vi "Calculate Average Center.vi"(11 "Gantry Fiducials":dbl[](array[numeric])) -> (3 "XYZTheta":dbl[](array[numeric]))   [LabVIEW 2020, in "Assembly Tray.lvclass"]
uses:
  Assembly Tray.lvclass
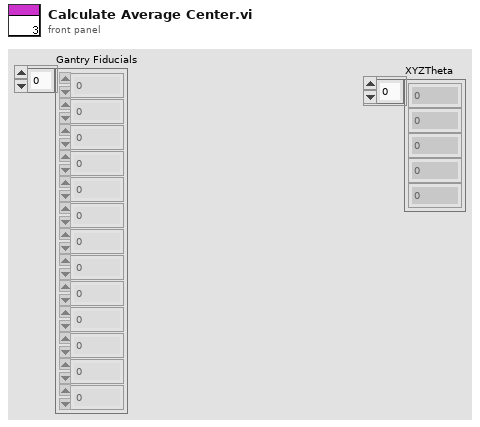
[diagram p1: front panel]
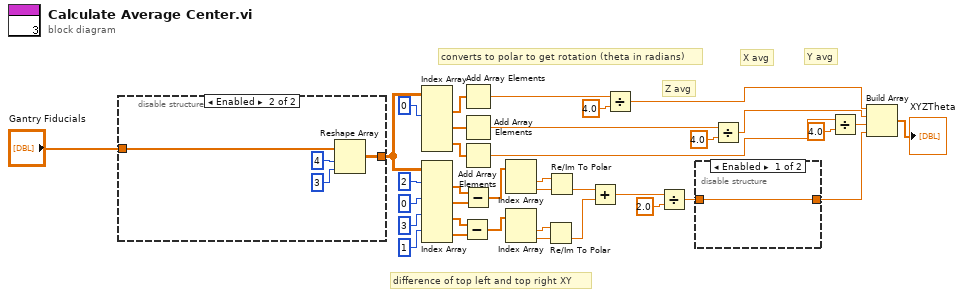
[diagram p0: block diagram]
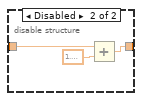
[diagram p2: hidden frame]
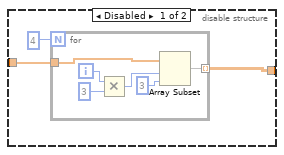
[diagram p3: hidden frame]
diagram:
  # "converts to polar to get rotation (theta in radians)"
  # "difference of top left and top right XY"
  # "Z avg"
  # "Y avg"
  # "X avg"
  n1 = disable-structure shown="Enabled" {
    disable-tunnel: [w39 w46] -> w4
    disable-tunnel: "Gantry Fiducials" -> [w37 w47]
    frame Disabled {
      n2 = for {
        N: 4 -> [_]
        tunnel: w37 -> [w41]
        tunnel: [w40] -> w39 mode=indexing
        i -> [w45]
        n3 = Multiply(x=w45, y=3) -> (x*y=w43:i32)
        n4 = Array Subset(array=w41, index=w43, length=3) -> (w40:dbl[])
      }
    }
    frame Enabled {
      n5 = Reshape Array(w47, 4 ("dimension size"), 3 ("dimension size")) -> (w46:dbl[][])
    }
  }
  n6 = Index Array(array=w4, index (col) #1=0 ("disabled index (col)")) -> (element #1=w33:dbl[], element #2=w32:dbl[], element #3=w3:dbl[])  [unwired: 5 in]
  n7 = Index Array(array=w4, index (row) #1=2 ("index (row)"), index (row) #2=0 ("index (row)"), index (row) #3=3 ("index (row)"), index (row) #4=1 ("index (row)")) -> (element #1=w17:dbl[], element #2=w16:dbl[], element #3=w15:dbl[], element #4=w14:dbl[])  [unwired: 4 in]
  n8 = Subtract(x=w15, y=w14) -> (x-y=w26:dbl[])
  n9 = Add Array Elements(numeric array=w33) -> (sum=w31:dbl)
  n10 = Add Array Elements(numeric array=w32) -> (sum=w30:dbl)
  n11 = Add Array Elements(numeric array=w3) -> (sum=w8:dbl)
  n12 = Subtract(x=w17, y=w16) -> (x-y=w27:dbl[])
  n13 = Index Array(array=w27) -> (element #1=w25:dbl, element #2=w24:dbl)  [unwired: 2 in]
  n14 = Index Array(array=w26) -> (element #1=w23:dbl, element #2=w22:dbl)  [unwired: 2 in]
  n15 = Re/Im To Polar(2:w22, 3:w23) -> (0:w20:dbl)  [unwired: 1 out]
  n16 = Re/Im To Polar(2:w24, 3:w25) -> (0:w21:dbl)  [unwired: 1 out]
  n17 = Add(x=w21, y=w20) -> (x+y=w19:dbl)
  n18 = Divide(x=w31, y=4.0) -> (x/y=w7:dbl)
  n19 = Divide(x=w19, y=2.0) -> (x/y=w2:dbl)
  n20 = disable-structure shown="Enabled" {
    disable-tunnel: w2 -> [w50 w52]
    disable-tunnel: [w50 w51] -> w1
    frame Enabled {
    }
    frame Disabled {
      n21 = Add(x=w52, y=1.5707963267948966) -> (x+y=w51:dbl)
    }
  }
  n22 = Divide(x=w30, y=4.0) -> (x/y=w6:dbl)
  n23 = Divide(x=w8, y=4.0) -> (x/y=w5:dbl)
  n24 = Build Array(w7, w6, w5, w1) -> (→"XYZTheta":dbl[])
